vi "get Ship Textures.vi"(11 "Ship in":refnum<class "Ship.lvclass">) -> (3 "Ship":string[](array[string]))   [LabVIEW 2021, in "Ship.lvclass"]
uses:
  Ship.lvclass
  Ship.lvclass/Ship.ctl
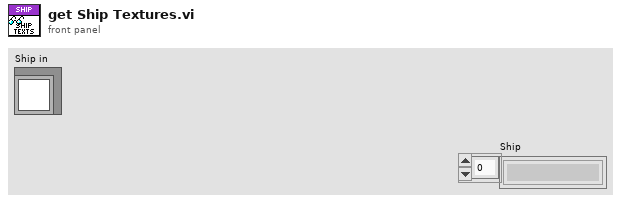
[diagram p1: front panel]
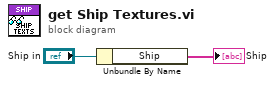
[diagram p0: block diagram]
diagram:
  n1 = Unbundle By Name("Ship in") -> ("Ship"=→"Ship":string[])
